vi "getApplicationState.vi"(8 "error in (no error)":errorcluster, 11 "VGS_RemoteControlClient in":refnum<class "VGS_RemoteControlClient.lvclass">) -> (0 "error out":errorcluster, 2 "getApplicationState":i32(ring)=1448165376 items=["NotRunning"=1448165376, "Starting"=1448165377, "Dying"=1448165378, "Idle"=1448165379, "WorkInProgress"=1448165380], 3 "VGS_RemoteControlClient out":refnum<class "VGS_RemoteControlClient.lvclass">)   [LabVIEW 2022 SP3, in "LV_VGS.lvlib" / "VGS_RemoteControlClient.lvclass"]
doc: "<B>Gets the current state of a VGStudio (MAX) instance. </B>\n\nThis method takes the remote handle and gets the current state of an application. The application can have one of the following states: NotRunning, Starting, Dying, Idle, WorkInProgress.\n\nParameters\nhandle A valid remote handle. \n\nEmit error RemoteControlServiceIsNotAvailableException if the remote control service doesn't run. \nEmit error GenericRemoteControlErrorException if an internal error occurs. \nEmit error InvalidRemoteHandleException if the remote handle is not valid."
uses:
  VGS_RemoteControlClient.lvclass
  VGS_RemoteControlClient.lvclass/VGS_RemoteControlClient.ctl
  C:/Users/Andrey/Documents/GitHub/LV_VGS/vgs_project.dll
  vgs_project.dll
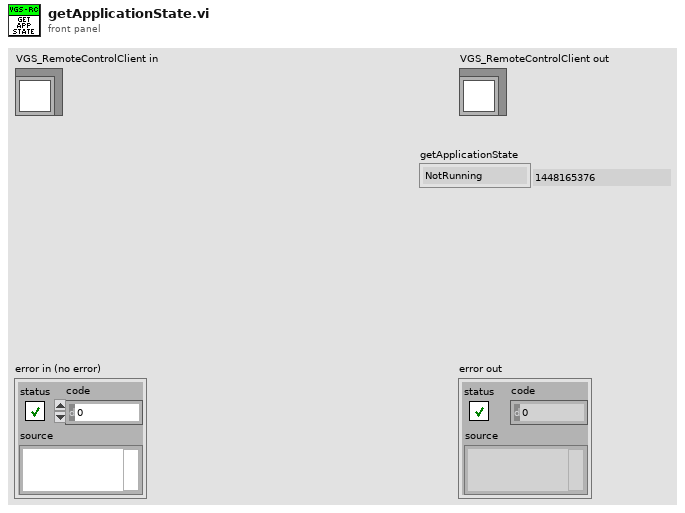
[diagram p1: front panel]
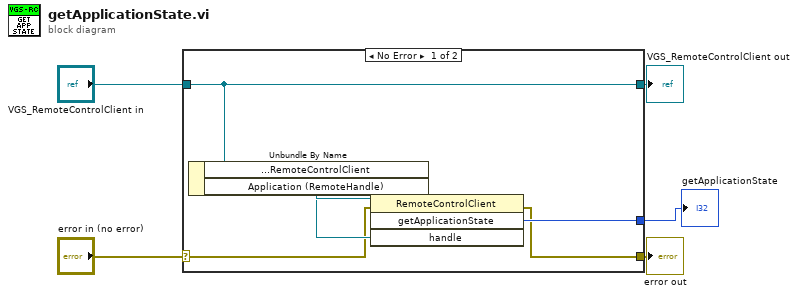
[diagram p0: block diagram]
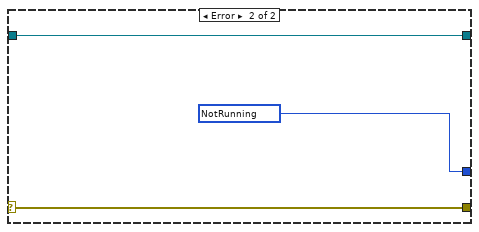
[diagram p2: hidden frame]
diagram:
  n1 = case shown="No Error" "error in (no error)" {
    selector: "error in (no error)" -> [w7 w13]
    tunnel: [w6 w13] -> w4
    tunnel: [w11 w14] -> w2
    tunnel: "VGS_RemoteControlClient in" -> [w11 w14]
    tunnel: [w8 w12] -> w1
    frame No Error {
      n2 = Unbundle By Name(w11) -> ("VGS.Project.Interop.RemoteControlClient"=w10:refnum<k24>, "Application (RemoteHandle)"=w9:refnum<k24>)
      n3 = invoke class="RemoteControlClient" method="getApplicationState"(reference=w10, error in=w7, "handle"=w9) -> (error out=w6:errorcluster, "getApplicationState"=w8:i32)  [unwired: 1 in, 2 out]
    }
    frame Error {
      w12 = 1448165376 items=["NotRunning"=1448165376, "Starting"=1448165377, "Dying"=1448165378, "Idle"=1448165379, "WorkInProgress"=1448165380] ("getApplicationState")
    }
  }
  "error out" <- w4
  "VGS_RemoteControlClient out" <- w2
  "getApplicationState" <- w1
